vi "FineReport_Select.vi"(7 "SelectColumn(array)":string[](array[string]), 8 "error in (no error)":errorcluster, 9 "SelectWhere":string, 10 "SelectTableName":string, 11 "ADODB._Connection in":refnum<k7>) -> (0 "error out":errorcluster, 1 "Rows Fetched":i32, 2 "OutData":string[][](array[string]), 3 "ADODB._Connection Out":refnum<k7>, 5 "有数据":bool)   [LabVIEW 2018]
panel:
  # "Rev2.0"
  # "Input"
  # "Output"
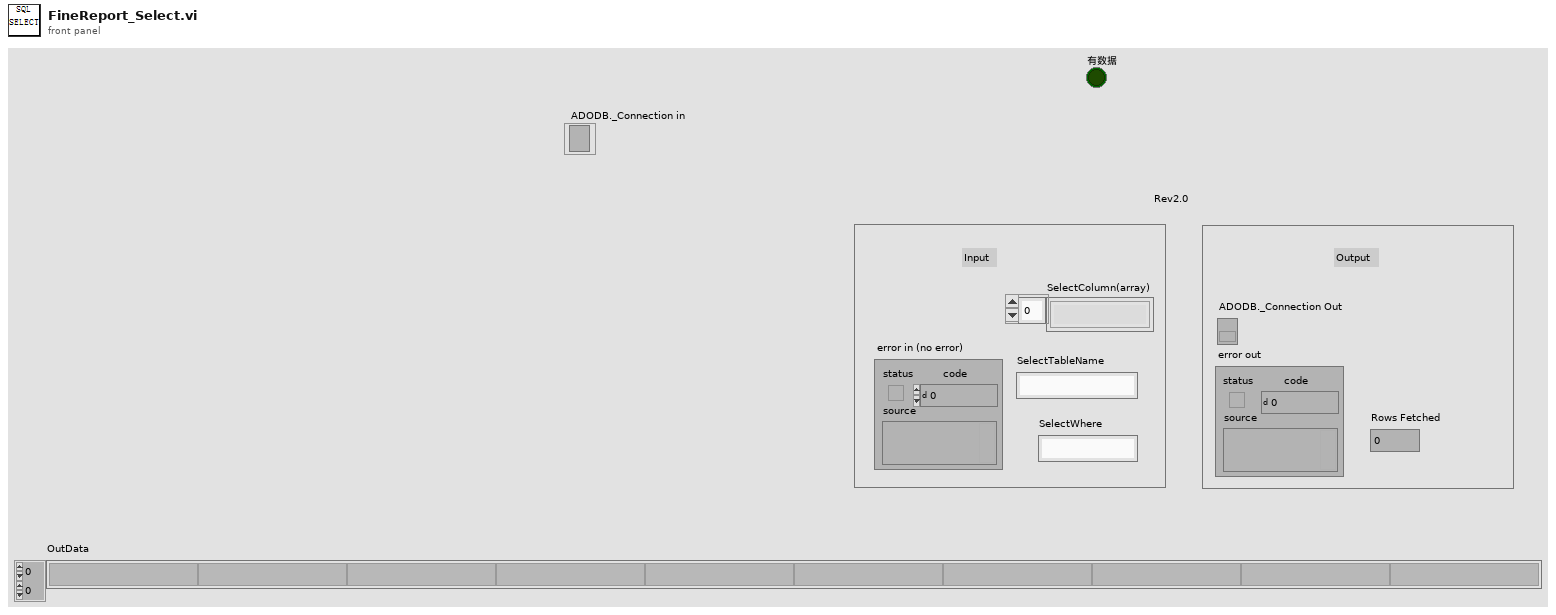
[diagram p1: front panel]
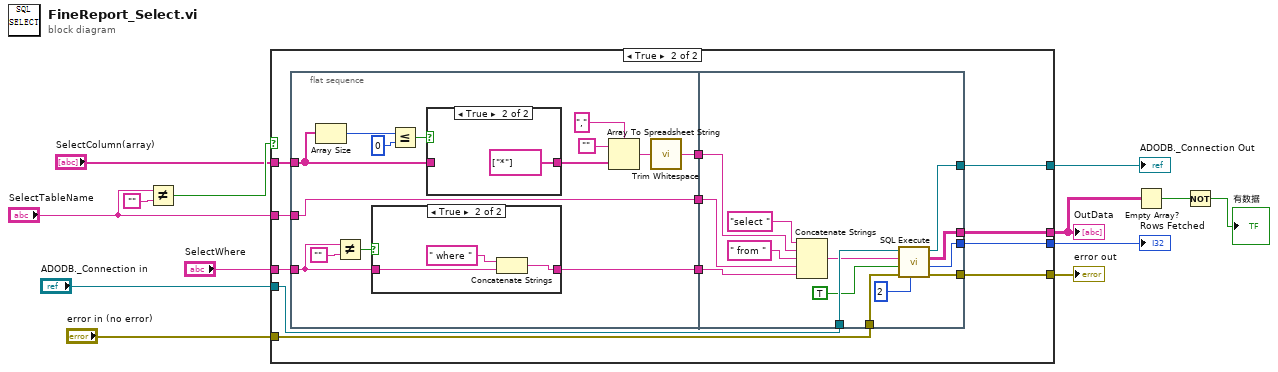
[diagram p0: block diagram]
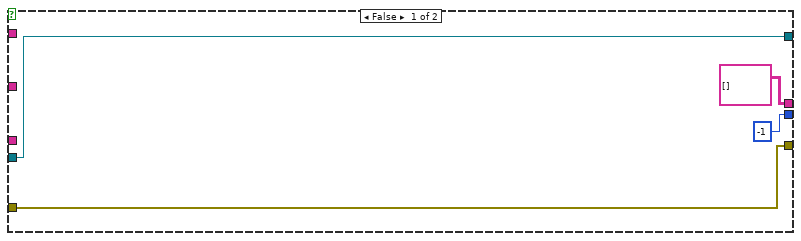
[diagram p2: hidden frame]
diagram:
  n1 = Not Equal?(x="SelectTableName", y="") -> (x != y?=w12:bool)
  n2 = case shown="True" w12 {
    tunnel: "ADODB._Connection in" -> [w17 w29]
    tunnel: "error in (no error)" -> [w16 w28]
    tunnel: [w17 w27] -> w7
    tunnel: [w16 w26] -> w6
    tunnel: "SelectColumn(array)" -> [_ w24]
    tunnel: "SelectWhere" -> [_ w22]
    tunnel: [string[][] [] ("Data") w21] -> w3
    tunnel: [-1 ("Rows Fetched") w20] -> w9
    tunnel: "SelectTableName" -> [_ w18]
    frame False {
    }
    frame True {
      n3 = flat-sequence {
        tunnel: [w34] -> w25
        tunnel: w24 -> [w37]
        tunnel: [w30] -> w23
        tunnel: w22 -> [w33]
        tunnel: [w32] -> w19
        tunnel: w18 -> [w32]
        tunnel: w29 -> [w63]
        tunnel: w28 -> [w62]
        tunnel: [w61] -> w27
        tunnel: [w60] -> w26
        tunnel: w25 -> [w51]
        tunnel: w23 -> [w55]
        tunnel: [w54] -> w21
        tunnel: [w53] -> w20
        tunnel: w19 -> [w52]
        frame #0 {
          n4 = Array Size(array=w37) -> (size(s)=w39:i32)
          n5 = Not Equal?(x=w33, y="") -> (x != y?=w42:bool)
          n6 = case shown="True" w42 {
            tunnel: [w46 w48] -> w34
            tunnel: w33 -> [w46 w47]
            frame False {
            }
            frame True {
              n7 = Concatenate Strings(" where " ("字符串"), w47) -> (w48:string)
            }
          }
          n8 = Less Or Equal?(x=w39, y=0) -> (x <= y?=w41:bool)
          n9 = case shown="True" w41 {
            tunnel: [w44 string[] ["*"] ("添加的数组 2")] -> w38
            tunnel: w37 -> [w44 _]
            frame False {
            }
            frame True {
            }
          }
          n10 = Array To Spreadsheet String(delimiter (Tab)="," ("分隔符(Tab)"), array=w38, 3:"" ("y")) -> (spreadsheet string=w31:string)
          n11 = call <vilib>:"Trim Whitespace.vi"("string"=w31) -> ("trimmed string"=w30:string)  [unwired: 1 in]
        }
        frame #1 {
          n12 = Concatenate Strings("select ", w55, " from " ("字符串"), w52, w51) -> (w58:string)
          n13 = call <userlib>:"SQL Execute.vi"("Retries"=2, "error in (no error)"=w62, "Return Data (T)"=TRUE, "Command Text"=w58, "ADODB._Connection In"=w63) -> ("error out"=w60:errorcluster, "Rows Fetched"=w53:i32, "Data"=w54:string[][], "ADODB._Connection Out"=w61:refnum<k7>)  [unwired: 3 in]
        }
      }
    }
  }
  "ADODB._Connection Out" <- w7
  "error out" <- w6
  "OutData" <- w3
  "Rows Fetched" <- w9
  n14 = Empty Array?(array=w3) -> (empty?=w2:bool)
  n15 = Not(x=w2) -> (.not. x?=→"有数据":bool)
